vi "API_RedElectrica.vi"() -> ()   [LabVIEW 2024]
uses:
  <vilib>/httpClient/LabVIEWHTTPClient.lvlib
panel:
  out "Precio + timestamp":cluster{"value":dbl, "datetime":string}[](array[cluster])
  out "concatenated string":string
  out "end_date":string
  out "start_date":string
  out "fecha_y_hora_con_un_dia_offset":string
  out "hora_actuall":string
  out "fecha y hora  actuales":string
  out "value":T1
  out "headers":string
  out "body":string
  # "VALORES DE SALIDA DEL JSON"
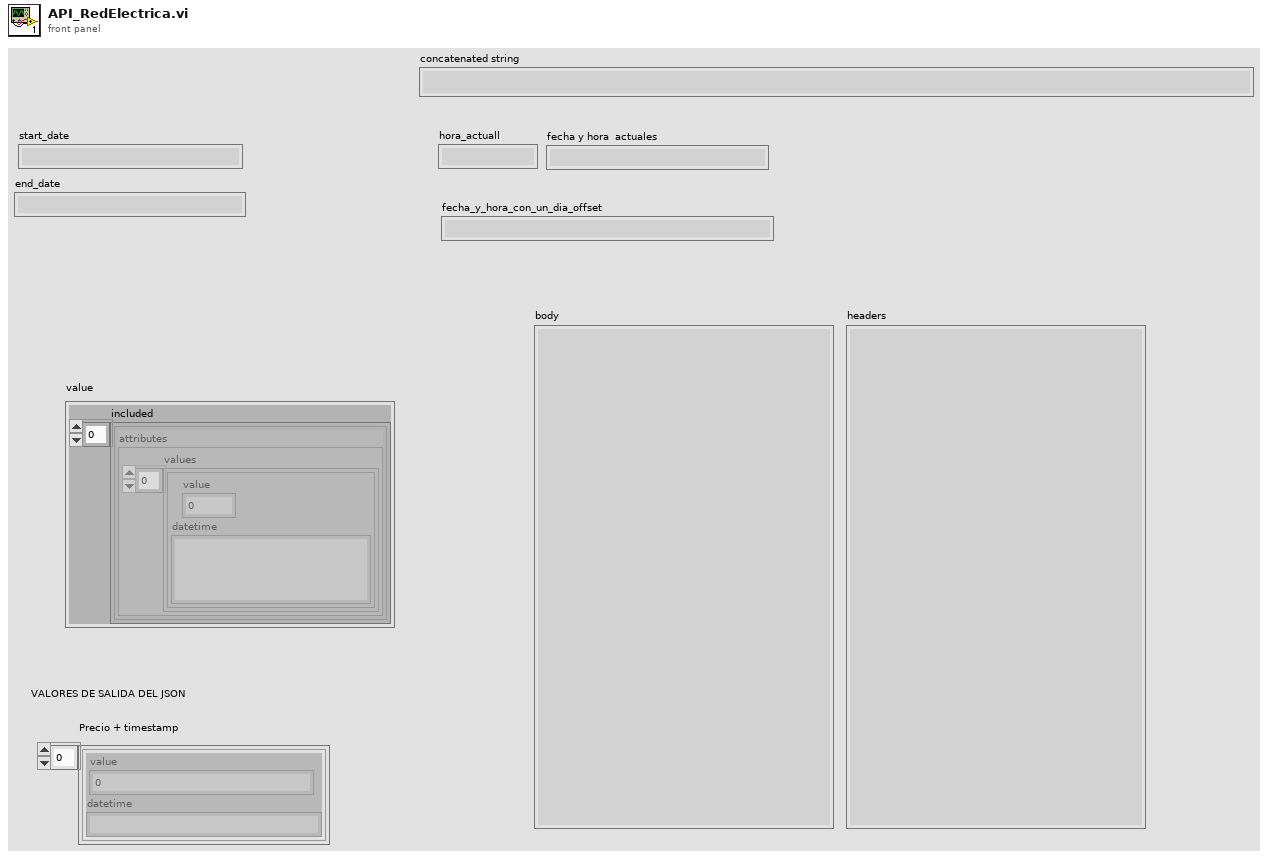
[diagram p1: front panel]
types:
  T1 = cluster{"included":cluster{"attributes":cluster{"values":cluster{"value":dbl, "datetime":string}[]}}[]}
  T2 = typedef "LabVIEWHTTPClient.lvlib/ClientHandle.ctl" = refnum<k1>
  T3 = cluster{"attributes":cluster{"values":cluster{"value":dbl, "datetime":string}[]}}[]
  T4 = cluster{"attributes":cluster{"values":cluster{"value":dbl, "datetime":string}[]}}
  T5 = cluster{"values":cluster{"value":dbl, "datetime":string}[]}
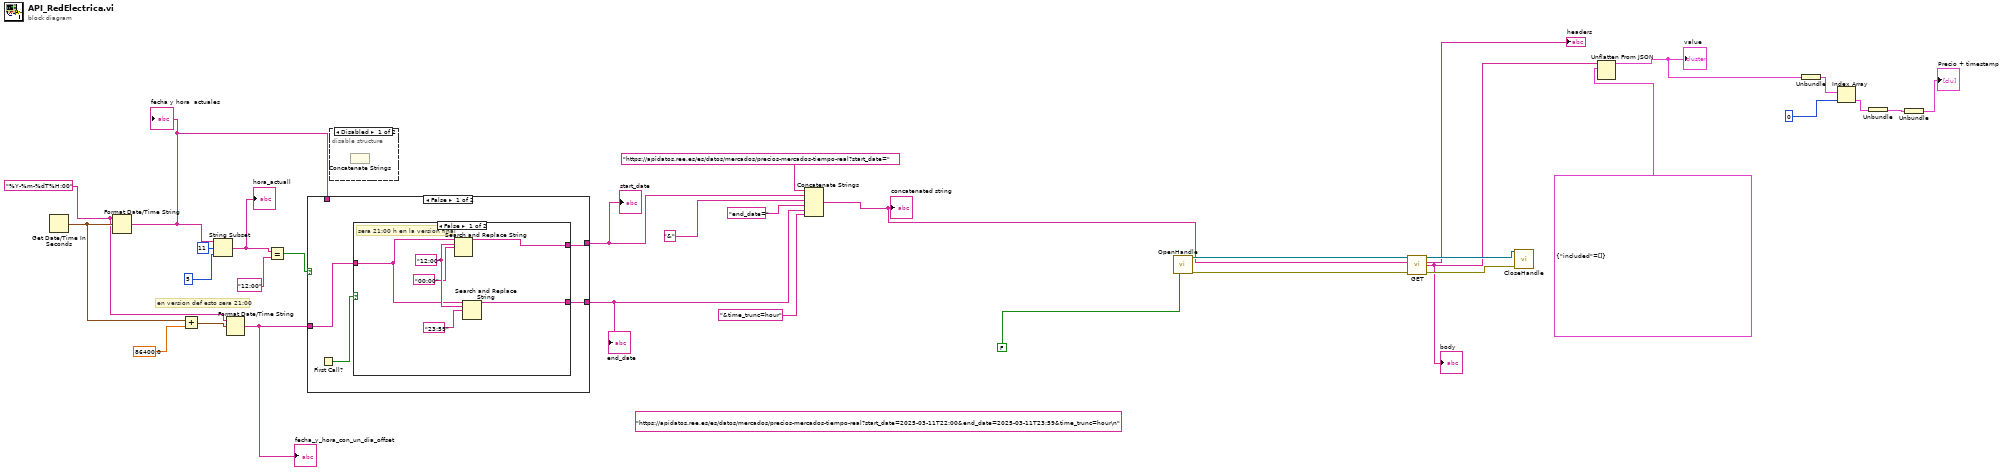
[diagram p0: block diagram]
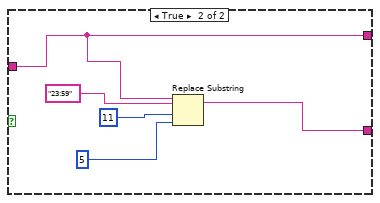
[diagram p3: hidden frame]
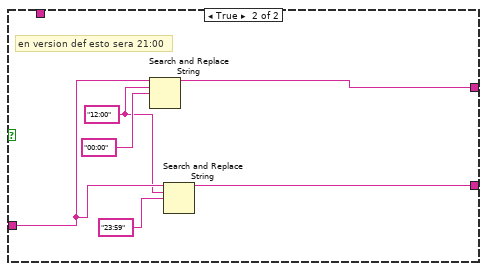
[diagram p4: hidden frame]
diagram:
  w11 = "%Y-%m-%dT%H:00" ("time format string (%c)")
  (unwired) "https://apidatos.ree.es/es/datos/mercados/precios-mercados-tiempo-real?start_date=2025-03-11T22:00&end_date=2025-03-11T23:59&time_trunc=hour\n" ("url")
  # "en version def esto sera 21:00"
  n1 = Get Date/Time In Seconds() -> (seconds since 1Jan1904=w14:timestamp)
  n2 = Format Date/Time String(time format string (%c)=w11, seconds (now)=w14) -> (date/time string=w9:string)  [unwired: 1 in]
  "fecha y hora  actuales" <- w9
  n3 = Add(x=w14, y=86400.0) -> (x+y=w12:timestamp)
  n4 = String Subset(string=w9, offset (0)=11, length (rest)=5 ("length (rest)")) -> (substring=w17:string)
  "hora_actuall" <- w17
  n5 = Format Date/Time String(time format string (%c)=w11, seconds (now)=w12) -> (date/time string=w10:string)  [unwired: 1 in]
  "fecha_y_hora_con_un_dia_offset" <- w10
  n6 = Equal?(x=w17, y="12:00") -> (x = y?=w15:bool)
  n7 = case shown="False" w15 {
    tunnel: w10 -> [w33 w52]
    tunnel: [w35 w49] -> w7
    tunnel: [w34 w48] -> w4
    tunnel: w9 -> [_ _]
    frame False {
      n8 = First Call?() -> (First Call?: T/F=w36:bool)
      n9 = case shown="False" w36 {
        tunnel: w33 -> [w39 w47]
        tunnel: [w37 w47] -> w35
        tunnel: [w38 w43] -> w34
        frame False {
          w42 = "12:00" ("search string")
          # "sera 21:00 h en la version final"
          n10 = Search and Replace String(input string=w39, search string=w42, replace string="00:00" ("replace string (\"\")")) -> (result string=w37:string)  [unwired: 5 in, 3 out]
          n11 = Search and Replace String(input string=w39, search string=w42, replace string="23:59" ("replace string (\"\")")) -> (result string=w38:string)  [unwired: 5 in, 3 out]
        }
        frame True {
          n12 = Replace Substring(2:5 ("length (len. of substring)"), 3:11 ("offset (0)"), 4:"23:59" ("substring (\"\")"), 5:w47) -> (1:w43:string)  [unwired: 1 out]
        }
      }
    }
    frame True {
      w51 = "12:00" ("search string")
      # "en version def esto sera 21:00"
      n13 = Search and Replace String(input string=w52, search string=w51, replace string="00:00" ("replace string (\"\")")) -> (result string=w49:string)  [unwired: 5 in, 3 out]
      n14 = Search and Replace String(input string=w52, search string=w51, replace string="23:59" ("replace string (\"\")")) -> (result string=w48:string)  [unwired: 5 in, 3 out]
    }
  }
  "start_date" <- w7
  "end_date" <- w4
  n15 = disable-structure shown="Disabled" {
    frame Disabled {
      n16 = Concatenate Strings() -> ()  [unwired: 2 in, 1 out]
    }
    frame Enabled {
    }
  }
  n17 = Concatenate Strings("https://apidatos.ree.es/es/datos/mercados/precios-mercados-tiempo-real?start_date=" ("string"), w7, "&" ("string"), "end_date=" ("string"), w4, "&time_trunc=hour" ("string")) -> (w2:string)
  "concatenated string" <- w2
  n18 = call <vilib>:"OpenHandle.vi"("verify server(true)"=FALSE) -> ("client handle out"=w32:T2, "error out"=w31:errorcluster)  [unwired: 13 in]
  n19 = call <vilib>:"GET.vi"("client handle"=w32, "url"=w2, "error in (no error)"=w31) -> ("client handle out"=w30:T2, "headers"=→"headers":string, "body"=w26:string, "error out"=w28:errorcluster)  [unwired: 9 in]
  "body" <- w26
  n20 = call <vilib>:"CloseHandle.vi"("client handle"=w30, "error in (no error)"=w28) -> ()  [unwired: 13 in, 1 out]
  n21 = Unflatten From JSON(JSON string=w26, type and defaults=T1 {"included"=[]}) -> (value=w24:T1)  [unwired: 5 in, 1 out]
  "value" <- w24
  n22 = Unbundle(w24) -> ("included"=w23:T3)
  n23 = Index Array(array=w23, index=0) -> (element=w21:T4)
  n24 = Unbundle(w21) -> ("attributes"=w20:T5)
  n25 = Unbundle(w20) -> ("values"=→"Precio + timestamp":cluster{"value":dbl, "datetime":string}[])
